vi "DeleteOldFiles.vi"(0 "object in":refnum<class "ErrorLogFile.lvclass">, 5 "Error In":errorcluster) -> (14 "object out":refnum<class "ErrorLogFile.lvclass">, 19 "Error Out":errorcluster)   [LabVIEW 2019, in "ErrorLogFile.lvclass"]
uses:
  ErrorLogFile.lvclass
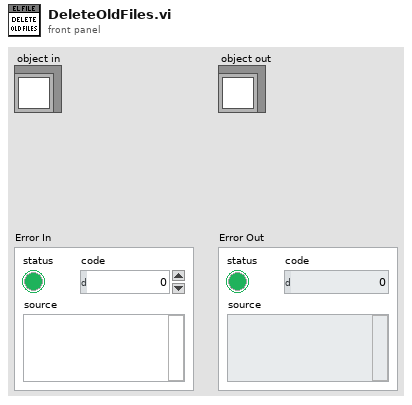
[diagram p1: front panel]
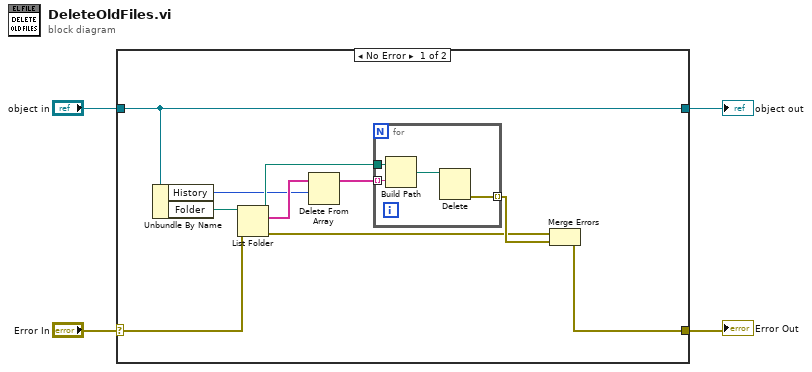
[diagram p0: block diagram]
diagram:
  n1 = case shown="No Error" "Error In" {
    selector: "Error In" -> [w7 w20]
    tunnel: [w6 w20] -> w3
    tunnel: [w14 w19] -> w1
    tunnel: "object in" -> [w14 w19]
    frame No Error {
      n2 = Unbundle By Name(w14) -> ("History"=w5:i32, "Folder"=w8:path)
      n3 = List Folder(path=w8, error in=w7) -> (path out=w13:path, filenames=w12:string[], error out=w9:errorcluster)  [unwired: 2 in, 1 out]
      n4 = Delete From Array(array=w12, length=w5) -> (array with subset deleted=w11:string[])  [unwired: 1 in, 1 out]
      n5 = for {
        tunnel: w13 -> [w18]
        tunnel: w11 -> [w17] mode=indexing
        tunnel: [w15] -> w10 mode=indexing
        n6 = Build Path(base path=w18, name or relative path=w17) -> (appended path=w16:path)
        n7 = Delete(path (use dialog)=w16) -> (error out=w15:errorcluster)  [unwired: 4 in, 2 out]
      }
      n8 = Merge Errors(w9, w10) -> (w6:errorcluster)
    }
    frame Error {
    }
  }
  "Error Out" <- w3
  "object out" <- w1
